vi "Reset Device Core.vi"(8 "error in (no error)":errorcluster, 11 "CS++SimMotor in":refnum<class "CS++SimMotor.lvclass">) -> (0 "error out":errorcluster, 3 "CS++SimMotor out":refnum<class "CS++SimMotor.lvclass">)   [LabVIEW 2015, in "CS++SimMotor.lvlib" / "CS++SimMotor.lvclass"]
doc: "Perform reset of device."
uses:
  CS++SimMotor.lvclass
  CS++SimMotor.lvclass/CS++SimMotor.ctl
  CSPP_DeviceBase/CS++Motor/CS++Motor.lvclass
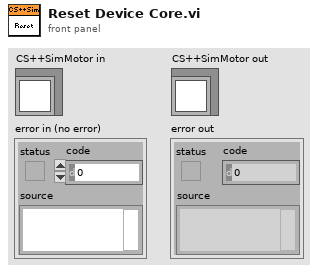
[diagram p1: front panel]
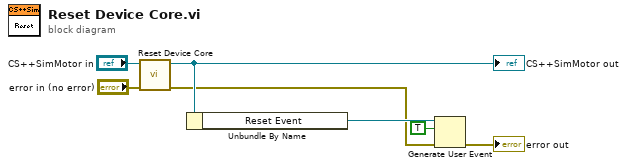
[diagram p0: block diagram]
diagram:
  n1 = call-parent "Reset Device Core.vi"("error in (no error)"="error in (no error)", "CS++Motor in"="CS++SimMotor in") -> ("error out"=w2:errorcluster, "CS++Motor out"=w5:refnum<class "CS++SimMotor.lvclass">)  [unwired: 8 in]
  "CS++SimMotor out" <- w5
  n2 = Unbundle By Name(w5) -> ("Reset Event"=w4:refnum<user-event>)
  n3 = Generate User Event(user event=w4, event data cluster=TRUE ("event data"), error in=w2) -> (error out=→"error out":errorcluster)  [unwired: 1 in, 1 out]
